vi "FTW-Endpoint-Core-RouterStart.vi"(0 "FTW Endpoint":refnum<class "FTW-Actor-Endpoint.lvclass">, 11 "error in":errorcluster) -> (4 "FTW Endpoint out":refnum<class "FTW-Actor-Endpoint.lvclass">, 6 "Incoming Message":refnum<event-registration>, 15 "error out":errorcluster)   [LabVIEW 2013, in "FTW-Actor-Endpoint.lvclass"]
uses:
  FTW-Actor-Endpoint.lvclass
  request/FTW-Request.lvclass
panel:
  # "Inputs"
  # "Outputs"
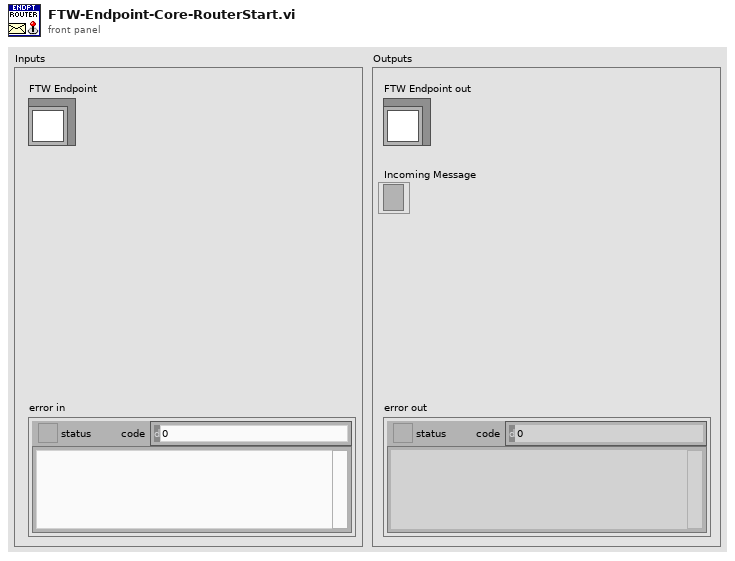
[diagram p1: front panel]
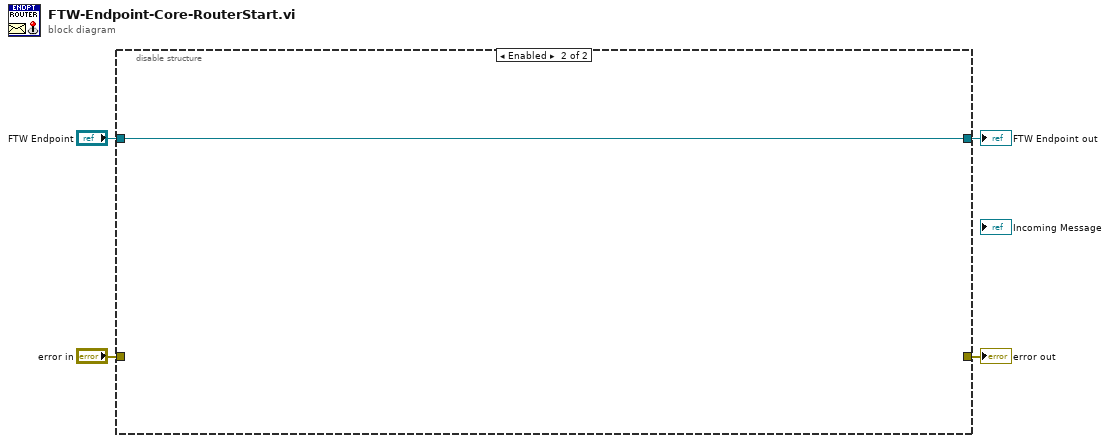
[diagram p0: block diagram]
diagram:
  n1 = disable-structure shown="Enabled" {
    disable-tunnel: [w8 _] -> w4
    disable-tunnel: "error in" -> [w7 _]
    disable-tunnel: "FTW Endpoint" -> [w6 w12]
    disable-tunnel: [w5 w12] -> w1
    frame Disabled {
      n2 = case shown="No Error" w7 {
        selector: w7 -> [_ w11]
        tunnel: [_ w11] -> w8
        tunnel: w6 -> [w9 w10]
        tunnel: [w9 w10] -> w5
        frame No Error {
        }
        frame Error {
        }
      }
    }
    frame Enabled {
    }
  }
  "error out" <- w4
  "FTW Endpoint out" <- w1
